vi "UART_online.vi"(6 "rst":bool, 8 "error in (no error)":errorcluster caption="错误输入（无错误）", 9 "baud rate (115200)":u32=115200 caption="波特率(115200)", 10 "地址":u8=1, 11 "BASE_COM":refnum<visa-resource-name>="COM1") -> (0 "error out":errorcluster caption="错误输出", 1 "retStr":string, 2 "OK":bool, 3 "BASE_COM_OUT":refnum<visa-resource-name>)   [LabVIEW 2015, in "UARTCOM.lvlib"]
uses:
  UARTCOM.lvlib
  <vilib>/Instr/_visa.llb/VISA Configure Serial Port (Instr).vi
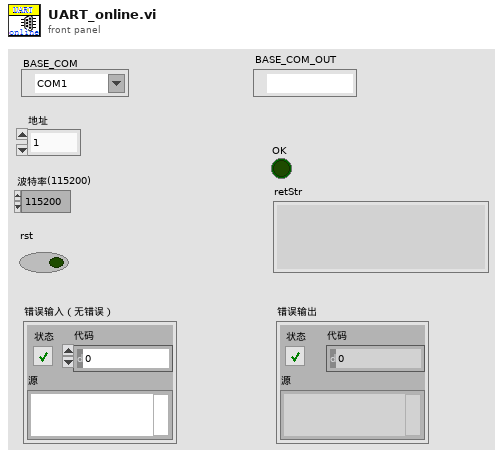
[diagram p1: front panel]
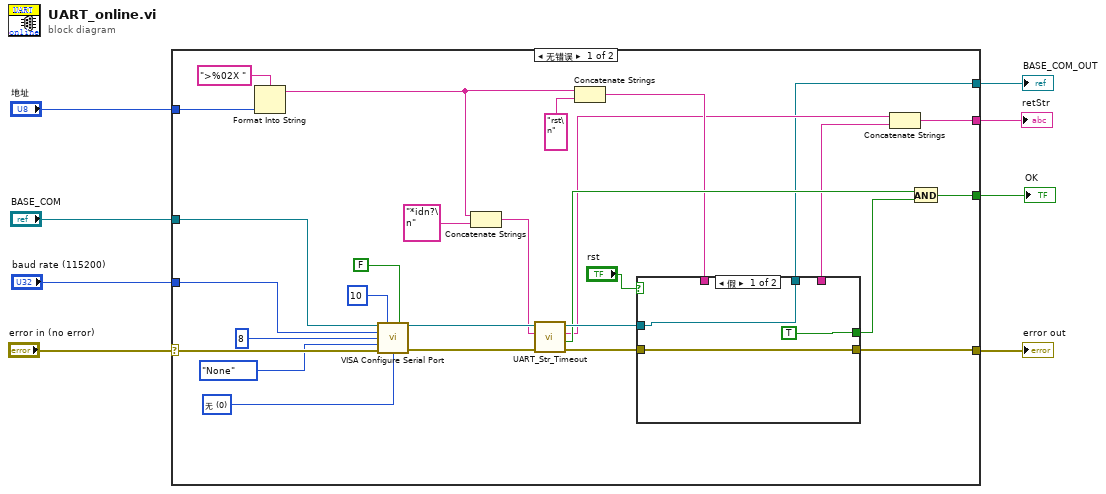
[diagram p0: block diagram]
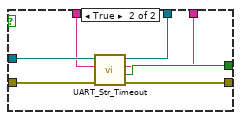
[diagram p2: hidden frame]
diagram:
  n1 = case shown="无错误" "error in (no error)" {
    selector: "error in (no error)" -> [w36 w48]
    tunnel: [w13 w48] -> w7
    tunnel: "BASE_COM" -> [w21 w47]
    tunnel: "baud rate (115200)" -> [w33 _]
    tunnel: [w22 _] -> w4
    tunnel: "地址" -> [w20 _]
    tunnel: [w10 _] -> w2
    tunnel: [w9 w47] -> w1
    frame No Error {
      w30 = u16 0 items=["无", "XON/XOFF", "RTS/CTS", "XON/XOFF & RTS/CTS", "DTR/DSR", "XON/XOFF & DTR/DSR"] ("flow control (0:none)")
      n2 = Format Into String(format string=">%02X ", w20) -> (resulting string=w15:string)  [unwired: 2 in, 1 out]
      n3 = call-poly "VISA Configure Serial Port"("VISA resource name"=w21, "timeout (10sec)"=u32 10, "Enable Termination\nChar (T)"=FALSE ("Enable Termination\nChar (T)"), "baud rate (9600)"=w33, "data bits (8)"=u16 8, "parity (0:none)"=enum16{"None", "Odd", "Even", "Mark", "Space"}."None", "error in (no error)"=w36, "flow control (0:none)"=w30) -> ("VISA resource name out"=w28:refnum<visa-resource-name>, "error out"=w29:errorcluster)  [unwired: 6 in]
      n4 = Concatenate Strings(w15, "*idn?\n" ("写入字符串")) -> (w17:string)
      n5 = call "UART_Str_Timeout.vi"("error in (no error)"=w29, "写入字符串"=w17, "BASE_COM"=w28) -> ("error out"=w26:errorcluster, "OK"=w23:bool, "读取字符串"=w12:string, "BASE_COM_OUT"=w27:refnum<visa-resource-name>)  [unwired: 4 in, 1 out]
      n6 = Concatenate Strings(w15, "rst\n" ("写入字符串")) -> (w14:string)
      n7 = case shown="假" "rst" {
        tunnel: w27 -> [w37 w46]
        tunnel: w26 -> [w39 w45]
        tunnel: [w39 w44] -> w13
        tunnel: [TRUE w43] -> w24
        tunnel: w14 -> [_ w42]
        tunnel: [_ w41] -> w11
        tunnel: [w37 w40] -> w9
        frame False {
        }
        frame True {
          n8 = call "UART_Str_Timeout.vi"("error in (no error)"=w45, "写入字符串"=w42, "BASE_COM"=w46) -> ("error out"=w44:errorcluster, "OK"=w43:bool, "读取字符串"=w41:string, "BASE_COM_OUT"=w40:refnum<visa-resource-name>)  [unwired: 4 in, 1 out]
        }
      }
      n9 = Concatenate Strings(w12, w11) -> (w10:string)
      n10 = And(x=w23, y=w24) -> (x .and. y?=w22:bool)
    }
    frame Error {
    }
  }
  "error out" <- w7
  "OK" <- w4
  "retStr" <- w2
  "BASE_COM_OUT" <- w1
